vi "Sweep Position.vi"(3 "Vsd Ramp Position":cluster{"Vsd On":dbl, "Vsd On Vg Dir":bool}, 4 "Direction":bool=TRUE, 5 "Vg Value (V)":dbl, 6 "Scan Values":T1={"Min Vg (V)"=0.0, "Max Vg (V)"=10.0, "Vm Start (V)"=5.0, "Vm Stop (V)"=9.0, "Steps/Sec"=100.0, "Vm Rate (Hz)"=100.0, "Wavelength Start (nm)"=450.0, "Wavelength Stop (nm)"=850.0, "Wavelength Step (nm)"=2.0, "Vsd (V)"=0.1, "Vg Step Size"=0.01, "Vsd Ramp Time (secs)"=0.1} {"Vsd Ramp Time (secs)" min=-10.0 max=10.0; "Vg Step Size" min=0.0 max=0.5; "Vsd (V)" min=-10.0 max=10.0; "Wavelength Step (nm)" min=0.0 max=500.0; "Wavelength Stop (nm)" min=16.0 max=2500.0; "Wavelength Start (nm)" min=15.0 max=2499.0; "Steps/Sec" min=1.0 max=1000.0; "Vm Stop (V)" min=-10.0 max=10.0; "Vm Start (V)" min=-10.0 max=10.0; "Max Vg (V)" min=-9.9 max=10.0; "Min Vg (V)" min=-10.0 max=9.9}) -> (0 "Recording":bool=TRUE, 1 "Vsd Ramp Sign":dbl, 2 "Start Vsd Ramp":bool=TRUE)   [LabVIEW 2009]
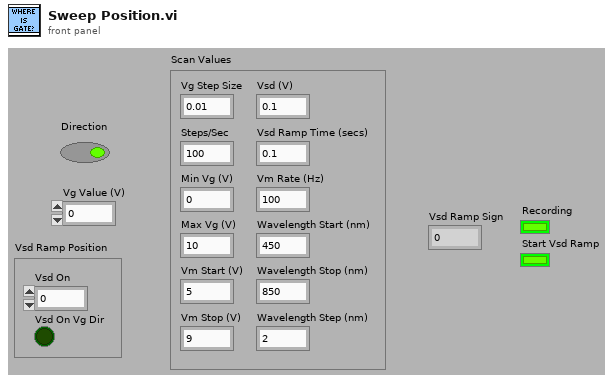
[diagram p1: front panel]
types:
  T1 = cluster{"Min Vg (V)":dbl, "Max Vg (V)":dbl, "Vm Start (V)":dbl, "Vm Stop (V)":dbl, "Steps/Sec":dbl, "Vm Rate (Hz)":dbl, "Wavelength Start (nm)":dbl, "Wavelength Stop (nm)":dbl, "Wavelength Step (nm)":dbl, "Vsd (V)":dbl, "Vg Step Size":dbl, "Vsd Ramp Time (secs)":dbl}
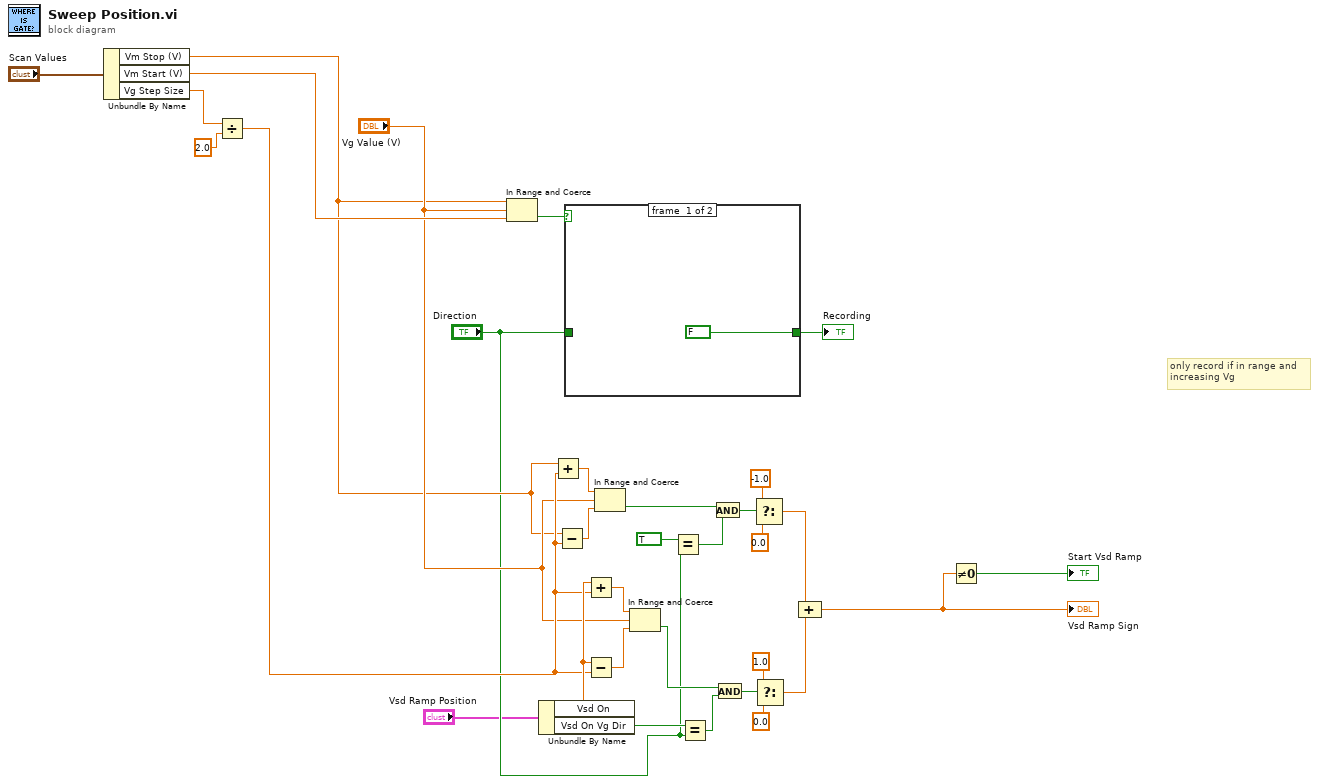
[diagram p0: block diagram]
diagram:
  # "only record if in range and\nincreasing Vg"
  n1 = Unbundle By Name("Scan Values") -> ("Vm Stop (V)"=w6:dbl, "Vm Start (V)"=w32:dbl, "Vg Step Size"=w29:dbl)
  n2 = Divide(x=w29, y=2.0) -> (x/y=w8:dbl)
  n3 = In Range and Coerce(upper limit=w6, x="Vg Value (V)", lower limit=w32) -> (In Range?=w30:bool)  [unwired: 1 out]
  n4 = Unbundle By Name("Vsd Ramp Position") -> ("Vsd On"=w11:dbl, "Vsd On Vg Dir"=w15:bool)
  n5 = Add(x=w6, y=w8) -> (x+y=w9:dbl)
  n6 = Subtract(x=w6, y=w8) -> (x-y=w10:dbl)
  n7 = case shown="False" w30 {
    tunnel: [FALSE w34] -> w31
    tunnel: "Direction" -> [_ w34]
    frame #0 {
    }
    frame #1 {
    }
  }
  "Recording" <- w31
  n8 = Add(x=w11, y=w8) -> (x+y=w13:dbl)
  n9 = Subtract(x=w11, y=w8) -> (x-y=w12:dbl)
  n10 = In Range and Coerce(upper limit=w9, x="Vg Value (V)", lower limit=w10) -> (In Range?=w19:bool)  [unwired: 1 out]
  n11 = In Range and Coerce(upper limit=w13, x="Vg Value (V)", lower limit=w12) -> (In Range?=w14:bool)  [unwired: 1 out]
  n12 = Equal?(x=TRUE, y="Direction") -> (x = y?=w18:bool)
  n13 = Equal?(x=w15, y="Direction") -> (x = y?=w16:bool)
  n14 = And(x=w19, y=w18) -> (x .and. y?=w20:bool)
  n15 = And(x=w14, y=w16) -> (x .and. y?=w21:bool)
  n16 = Select(t=-1.0 ("Vsd Ramp Sign"), s=w20, f=0.0 ("Vsd Ramp Sign")) -> (s? t:f=w27:dbl)
  n17 = Select(t=1.0 ("Vsd Ramp Sign"), s=w21, f=0.0 ("Vsd Ramp Sign")) -> (s? t:f=w26:dbl)
  n18 = Compound Arithmetic op=ADD(w27, w26) -> (w3:dbl)
  "Vsd Ramp Sign" <- w3
  n19 = Not Equal To 0?(x=w3) -> (x != 0?=→"Start Vsd Ramp":bool)
